vi "Mice Folder.vi"() -> (3 "Mice Folder":path)   [LabVIEW 2020, in "App.lvlib" / "MazeUI.lvclass"]
uses:
  MazeUI.lvclass
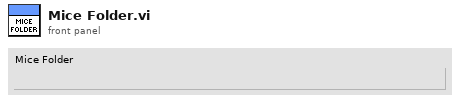
[diagram p1: front panel]
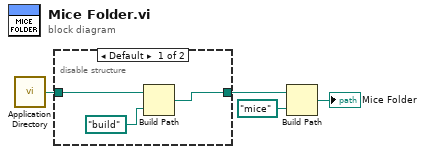
[diagram p0: block diagram]
diagram:
  n1 = call <vilib>:"Application Directory.vi"() -> ("Application Directory"=w3:path)
  n2 = disable-structure shown="Default" {
    disable-tunnel: w3 -> [w5 w8]
    disable-tunnel: [w6 w8] -> w2
    frame condition #0 (active) {
      n3 = Build Path(base path=w5, name or relative path=path "build") -> (appended path=w6:path)
    }
    frame condition #1 {
    }
  }
  n4 = Build Path(base path=w2, name or relative path=path "mice") -> (appended path=→"Mice Folder":path)
